vi "Teleop - Control Panel(SubVI).vi"(1 "Constant Cluster":T1 {"32. shooterHoodAngleRange" format="%_6f"; "31. turretAngleRange" format="%_6f"; "30. shooterVelocityLowerLimit" format="%_6f"; "29. shooterVelocityUpperLimit" format="%_6f"; "28. Robot Track Width (inches)" format="%_6f"; "27. Shooter Spin Up Speed (RPM)" format="%_6f"; "26. Climb Down Speed %" format="%_6f"; "25. Climb Up Speed %" format="%_6f"; "24. wallShooterVelocity" format="%_6f"; "23. Intake Spit Speed %" format="%_6f"; "22. Intake Suck Speed %" format="%_6f"; "21. CP Wheel Diameter" format="%_6f"; "20. Clockwise CP Fudge" format="%_6f"; "19. CouterClockwise CP Fudge" format="%_6f"; "18. Inches per Sector" format="%_6f"; "17. Ticks/Rotation Neo 550" format="%_6f"; "16. Control Panel Wheel Diameter" format="%_6f"; "15. Center-Center Sector Distance" format="%_6f"; "14. Inches / Tick Drivetrain" format="%_6f"; "13. Auton I Output Limit Drive Straight Gain" format="%_6f"; "12. Auton Deriv Drive Straight Gain" format="%_6f"; "11. Auton Int Drive Straight Gain" format="%_6f"; "10. Auton Prop Drive Straight Gain" format="%_6f"; "9. Auton I Output Limit Turn Gain" format="%_6f"; "8. Auton Deriv Turn Gain" format="%_6f"; "7. Auton Int Turn Gain" format="%_6f"; "1. Auton Prop Drive Gain" format="%_6f"; "2. Auton Int Drive Gain" format="%_6f"; "3. Auton Deriv Drive Gain" format="%_6f"; "4. I Output Drive  Limit" format="%_6f"; "5. Auto Drive Cheat (%)" format="%_6f"; "6. Auton Prop Turn Gain" format="%_6f"}, 3 "disabled":bool, 5 "Game Specific Data":string, 7 "Matched Color Name":string, 9 "Raise / Lower Cylinder":bool, 11 "Rotate to Game Color":bool, 12 "Rotate 3-5 Times":bool) -> (2 "colorWheelOut":bool, 4 "controlPanelCylinder":enum16{"off", "on", "forward", "back"}(ring), 6 "Ticks to Move":dbl)   [LabVIEW 2019]
uses:
  Disabled/Constant VI_s/Disabled - Constant Cluster Typedef.ctl
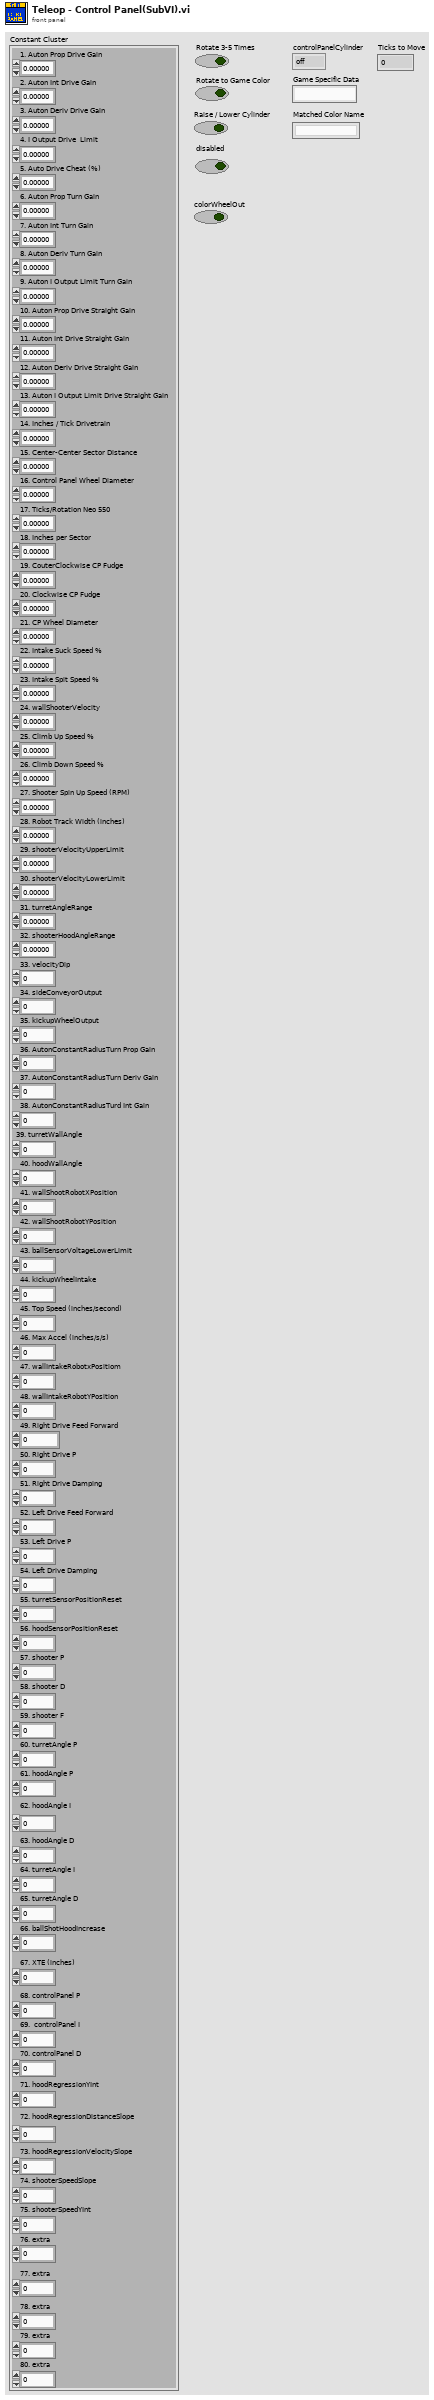
[diagram p1: front panel]
types:
  T1 = typedef "Disabled - Constant Cluster Typedef.ctl" = cluster{"1. Auton Prop Drive Gain":dbl, "2. Auton Int Drive Gain":dbl, "3. Auton Deriv Drive Gain":dbl, "4. I Output Drive  Limit":dbl, "5. Auto Drive Cheat (%)":dbl, "6. Auton Prop Turn Gain":dbl, "7. Auton Int Turn Gain":dbl, "8. Auton Deriv Turn Gain":dbl, "9. Auton I Output Limit Turn Gain":dbl, "10. Auton Prop Drive Straight Gain":dbl, "11. Auton Int Drive Straight Gain":dbl, "12. Auton Deriv Drive Straight Gain":dbl, "13. Auton I Output Limit Drive Straight Gain":dbl, "14. Inches / Tick Drivetrain":dbl, "15. Center-Center Sector Distance":dbl, "16. Control Panel Wheel Diameter":dbl, "17. Ticks/Rotation Neo 550":dbl, "18. Inches per Sector":dbl, "19. CouterClockwise CP Fudge":dbl, "20. Clockwise CP Fudge":dbl, "21. CP Wheel Diameter":dbl, "22. Intake Suck Speed %":dbl, "23. Intake Spit Speed %":dbl, "24. wallShooterVelocity":dbl, "25. Climb Up Speed %":dbl, "26. Climb Down Speed %":dbl, "27. Shooter Spin Up Speed (RPM)":dbl, "28. Robot Track Width (inches)":dbl, "29. shooterVelocityUpperLimit":dbl, "30. shooterVelocityLowerLimit":dbl, "31. turretAngleRange":dbl, "32. shooterHoodAngleRange":dbl, "33. velocityDip":dbl, "34. sideConveyorOutput":dbl, "35. kickupWheelOutput":dbl, "36. AutonConstantRadiusTurn Prop Gain":dbl, "37. AutonConstantRadiusTurn Deriv Gain":dbl, "38. AutonConstantRadiusTurd Int Gain":dbl, "39. turretWallAngle":dbl, "40. hoodWallAngle":dbl, "41. wallShootRobotXPosition":dbl, "42. wallShootRobotYPosition":dbl, "43. ballSensorVoltageLowerLimit":dbl, "44. kickupWheelIntake":dbl, "45. Top Speed (inches/second)":dbl, "46. Max Accel (inches/s/s)":dbl, "47. wallIntakeRobotxPositiom":dbl, "48. wallIntakeRobotYPosition":dbl, "49. Right Drive Feed Forward":dbl, "50. Right Drive P":dbl, "51. Right Drive Damping":dbl, "52. Left Drive Feed Forward":dbl, "53. Left Drive P":dbl, "54. Left Drive Damping":dbl, "55. turretSensorPositionReset":dbl, "56. hoodSensorPositionReset":dbl, "57. shooter P":dbl, "58. shooter D":dbl, "59. shooter F":dbl, "60. turretAngle P":dbl, "61. hoodAngle P":dbl, "62. hoodAngle I":dbl, "63. hoodAngle D":dbl, "64. turretAngle I":dbl, "65. turretAngle D":dbl, "66. ballShotHoodIncrease":dbl, "67. XTE (inches)":dbl, "68. controlPanel P":dbl, "69.  controlPanel I":dbl, "70. controlPanel D":dbl, "71. hoodRegressionYInt":dbl, "72. hoodRegressionDistanceSlope":dbl, "73. hoodRegressionVelocitySlope":dbl, "74. shooterSpeedSlope":dbl, "75. shooterSpeedYInt":dbl, "76. extra":dbl, "77. extra":dbl, "78. extra":dbl, "79. extra":dbl, "80. extra":dbl}
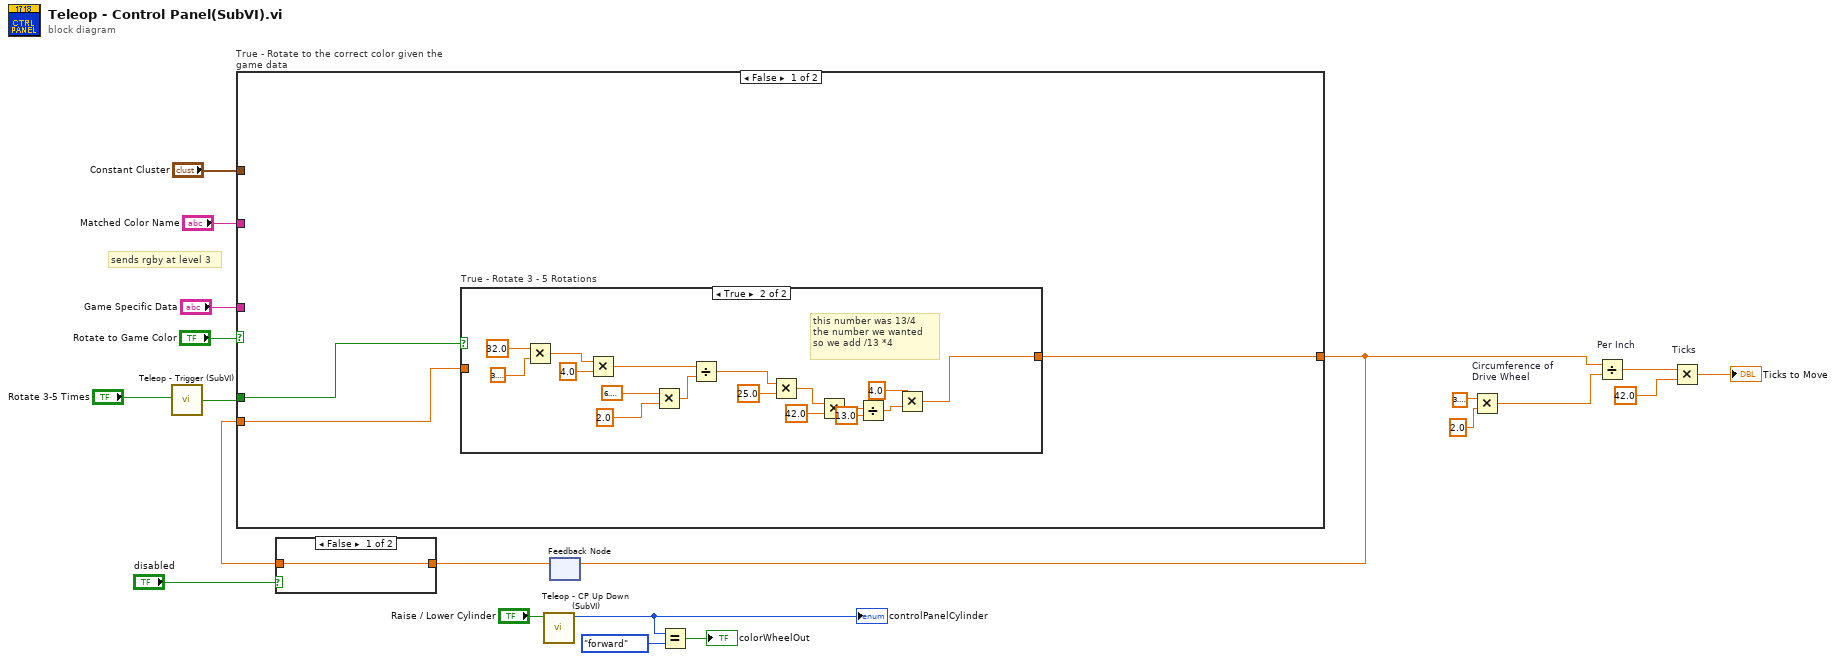
[diagram p0: block diagram]
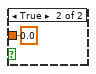
[diagram p2: hidden frame]
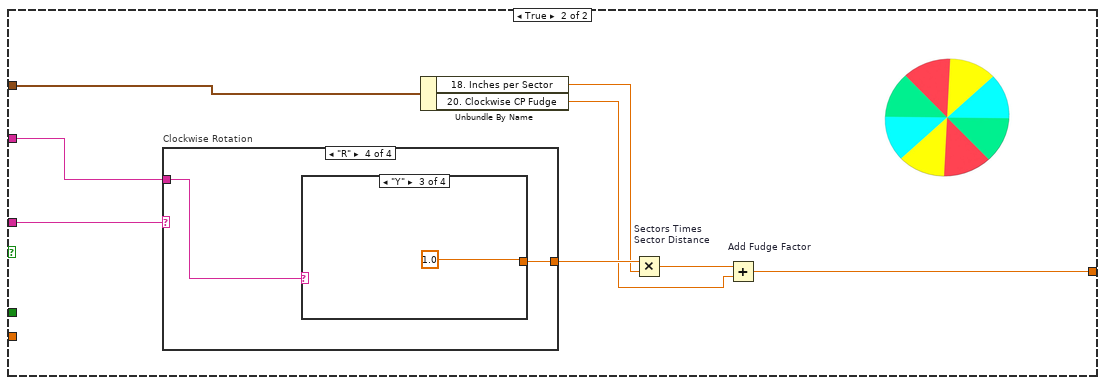
[diagram p4: hidden frame]
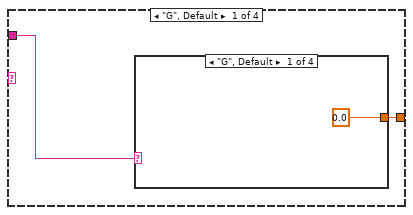
[diagram p5: hidden frame]
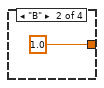
[diagram p6: hidden frame]
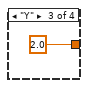
[diagram p7: hidden frame]
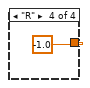
[diagram p8: hidden frame]
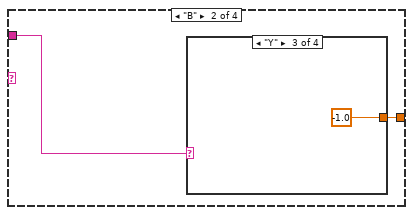
[diagram p9: hidden frame]
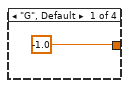
[diagram p10: hidden frame]
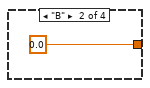
[diagram p11: hidden frame]
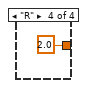
[diagram p12: hidden frame]
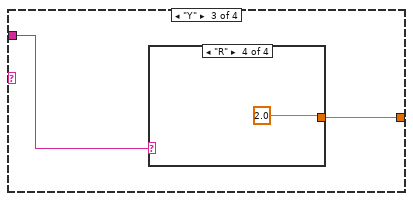
[diagram p13: hidden frame]
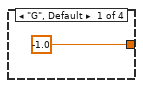
[diagram p14: hidden frame]
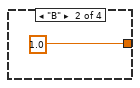
[diagram p15: hidden frame]
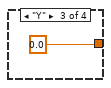
[diagram p16: hidden frame]
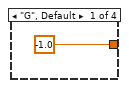
[diagram p17: hidden frame]
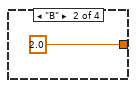
[diagram p18: hidden frame]
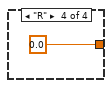
[diagram p19: hidden frame]
diagram:
  # "sends rgby at level 3"
  n1 = call "Teleop - Trigger (SubVI).vi"("Trigger"="Rotate 3-5 Times") -> ("Trigger Output"=w4:bool)
  n2 = call "Teleop - CP Up Down (SubVI).vi"("Raise / Lower Cylinder"="Raise / Lower Cylinder") -> ("controlPanelCylinder"=w3:enum16{"off", "on", "forward", "back"})  [unwired: 10 in]
  "controlPanelCylinder" <- w3
  n3 = feedback #1() -> (w7:dbl)  [unwired: 1 in]
  n4 = case shown="False" "disabled" {
    tunnel: w7 -> [w21 _]
    tunnel: [w21 0.0] -> w6
    frame False {
    }
    frame True {
    }
  }
  n5 = case "True - Rotate to the correct color given the game data" shown="False" "Rotate to Game Color" {
    tunnel: "Game Specific Data" -> [_ w49]
    tunnel: "Matched Color Name" -> [_ w48]
    tunnel: [w24 w44] -> w12
    tunnel: w6 -> [w25 _]
    tunnel: w4 -> [w23 _]
    tunnel: "Constant Cluster" -> [_ w45]
    frame False {
      n6 = case "True - Rotate 3 - 5 Rotations" shown="True" w23 {
        tunnel: [w26 w27] -> w24
        tunnel: w25 -> [w26 _]
        frame False {
        }
        frame True {
          # "this number was 13/4 \nthe number we wanted \nso we add /13 *4"
          n7 = Multiply(x=32.0, y=3.141592653589793) -> (x*y=w42:dbl)
          n8 = Multiply(x=w42, y=4.0) -> (x*y=w40:dbl)
          n9 = Multiply(x=6.283185307179586, y=2.0) -> (x*y=w36:dbl)
          n10 = Divide(x=w40, y=w36) -> (x/y=w35:dbl)
          n11 = Multiply(x=w35, y=25.0) -> (x*y=w32:dbl)
          n12 = Multiply(x=w32, y=42.0) -> (x*y=w31:dbl)
          n13 = Divide(x=w31, y=13.0) -> (x/y=w29:dbl)
          n14 = Multiply(x=4.0, y=w29) -> (x*y=w27:dbl)
        }
      }
    }
    frame True {
      n15 = case "Clockwise Rotation" shown="\"R\"" w49 {
        tunnel: w48 -> [w53 w59 w65 w71]
        tunnel: [w52 w58 w64 w70] -> w51
        frame "G", Default {
          n16 = case shown="\"G\", Default" w53 {
            tunnel: [0.0 ("controlPanelPosition") 1.0 ("controlPanelPosition") 2.0 ("controlPanelPosition") -1.0 ("controlPanelPosition")] -> w52
            frame "G", Default {
            }
            frame "B" {
            }
            frame "Y" {
            }
            frame "R" {
            }
          }
        }
        frame "B" {
          n17 = case shown="\"Y\"" w59 {
            tunnel: [-1.0 ("controlPanelPosition") 0.0 ("controlPanelPosition") -1.0 ("controlPanelPosition") 2.0 ("controlPanelPosition")] -> w58
            frame "G", Default {
            }
            frame "B" {
            }
            frame "Y" {
            }
            frame "R" {
            }
          }
        }
        frame "Y" {
          n18 = case shown="\"R\"" w65 {
            tunnel: [-1.0 ("controlPanelPosition") 1.0 ("controlPanelPosition") 0.0 ("controlPanelPosition") 2.0 ("controlPanelPosition")] -> w64
            frame "G", Default {
            }
            frame "B" {
            }
            frame "Y" {
            }
            frame "R" {
            }
          }
        }
        frame "R" {
          n19 = case shown="\"Y\"" w71 {
            tunnel: [-1.0 ("controlPanelPosition") 2.0 ("controlPanelPosition") 1.0 ("controlPanelPosition") 0.0 ("controlPanelPosition")] -> w70
            frame "G", Default {
            }
            frame "B" {
            }
            frame "Y" {
            }
            frame "R" {
            }
          }
        }
      }
      n20 = Unbundle By Name(w45) -> ("18. Inches per Sector"=w46:dbl, "20. Clockwise CP Fudge"=w47:dbl)
      n21 = Multiply "Sectors Times\nSector Distance"(x=w51, y=w46) -> (x*y=w50:dbl)
      n22 = Add "Add Fudge Factor"(x=w50, y=w47) -> (x+y=w44:dbl)
    }
  }
  n23 = feedback-in #1(w12) -> ()
  n24 = Equal?(x=w3, y=enum16{"off", "on", "forward", "back"}."forward") -> (x = y?=→"colorWheelOut":bool)
  n25 = Multiply "Circumference of\nDrive Wheel"(x=3.141592653589793, y=2.0) -> (x*y=w14:dbl)
  n26 = Divide "Per Inch"(x=w12, y=w14) -> (x/y=w17:dbl)
  n27 = Multiply "Ticks"(x=w17, y=42.0) -> (x*y=→"Ticks to Move":dbl)
